vi "Test Functionality.vi"() -> ()   [LabVIEW 2013, in "Exponential Fit Library.lvlib" / "Fit Exponential.lvclass"]
doc: "This is a simle demonstration of the capabilities of the exponential fit class."
uses:
  Fit Exponential.lvclass
  Fit Exponential.lvclass/Fit Exponential.ctl
  Children/DFT-1/DFT-1.lvclass
  Children/DFT-5/DFT-5.lvclass
  Children/LRS/LRS.lvclass
  Read Output.vi
  <vilib>/Analysis/1siggen.llb/Ramp Pattern by Delta.vi
  <vilib>/Analysis/NI_AALBase.lvlib
panel:
  out "Fit Output":T1
  in  "B":dbl
  in  "A":dbl
  in  "tau":dbl
  in  "Select Method":enum8{"DFT-1", "DFT-5", "LRS"}(ring)=enum."LRS"
  out "Error in Tau":dbl(graph)
  out "Tau":dbl(graph)
  out "Exponential":dbl[](graph)
  # "Exponential Input"
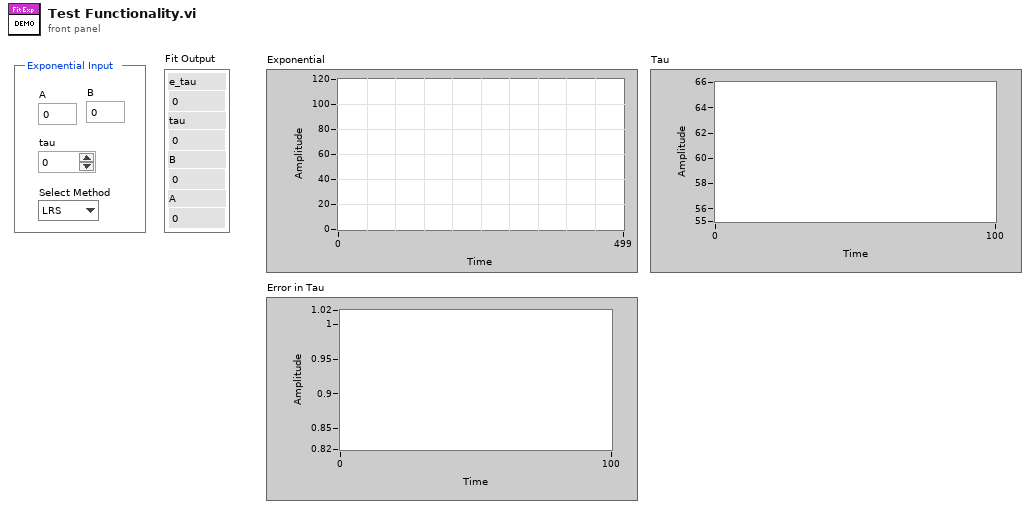
[diagram p1: front panel]
types:
  T1 = cluster{"e_tau":dbl, "tau":dbl, "B":dbl, "A":dbl}
  T2 = cluster{"A":dbl, "B":dbl, "tau":dbl, "e_tau":dbl}
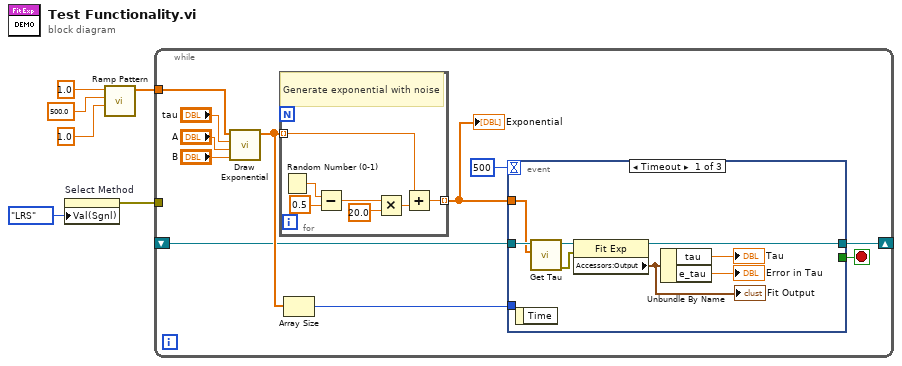
[diagram p0: block diagram]
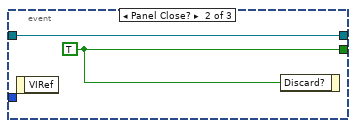
[diagram p2: hidden frame]
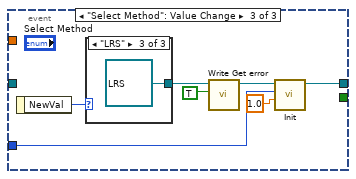
[diagram p3: hidden frame]
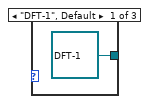
[diagram p4: hidden frame]
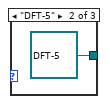
[diagram p5: hidden frame]
diagram:
  n1 = property on="Select Method" class="Enum (strict)"("Val(Sgnl)"=enum8{"DFT-1", "DFT-5", "LRS"}."LRS" ("Value (Signaling)")) -> (error out=w1:errorcluster)  [unwired: 2 in, 1 out]
  n2 = call-poly <vilib>:"Ramp Pattern.vi"("start"=1.0, "end"=500.0, "delta"=1.0) -> ("Ramp Pattern"=w3:dbl[])  [unwired: 6 in, 2 out]
  n3 = while {
    tunnel: w3 -> [w17]
    shift-right: [w13] -> _
    shift-left: _ -> [w9]
    tunnel: w1 -> [_]
    stop <- w7 stop-if-true
    n4 = call "Draw Exponential.vi"("B"="B", "A"="A", "tau"="tau", "time"=w17) -> ("ExponentialOut"=w12:dbl[])  [unwired: 7 in]
    n5 = for {
      tunnel: w12 -> [w39] mode=indexing
      tunnel: [w38] -> w8 mode=indexing
      # "Generate exponential with noise"
      n6 = Random Number (0-1)() -> (number: 0 to 1=w44:dbl)
      n7 = Subtract(x=w44, y=0.5) -> (x-y=w42:dbl)
      n8 = Multiply(x=w42, y=20.0) -> (x*y=w40:dbl)
      n9 = Add(x=w39, y=w40) -> (x+y=w38:dbl)
    }
    "Exponential" <- w8
    n10 = Array Size(array=w12) -> (size(s)=w11:i32)
    n11 = event shown="[0] Timeout" {
      selector: _ -> [_ _ _]
      dyn-events: _ -> [_ _ _]
      timeout: 500 -> [_ _ _]
      tunnel: [w22 w26 w33] -> w13
      tunnel: w11 -> [_ _ w32]
      tunnel: w9 -> [w25 w26 _]
      tunnel: w8 -> [w21 _ _]
      tunnel: [_ w27 _] -> w7
      event Timeout {
        n12 = event-data() -> ()  [unwired: 1 in, 1 out]
        n13 = call "Get Tau.vi"("Data In"=w21, "Fit Exp in"=w25) -> ("error out"=w23:errorcluster, "Fit Exp out"=w24:refnum<class "Fit Exponential.lvclass">)  [unwired: 8 in]
        n14 = property class="Fit Exp"(reference=w24, error in=w23) -> (reference out=w22:refnum<class "Fit Exponential.lvclass">, "Accessors:Output"=w18:T2)  [unwired: 1 out]
        "Fit Output" <- w18
        n15 = Unbundle By Name(w18) -> ("tau"=→"Tau":dbl, "e_tau"=→"Error in Tau":dbl)
      }
      event Panel Close? {
        w27 = TRUE
        n16 = event-data() -> ()  [unwired: 1 in, 1 out]
        n17 = event-data("Discard?"=w27) -> ()  [unwired: 1 in, 1 out]
      }
      event "Select Method": Value Change {
        n18 = event-data() -> ("NewVal"=w34:enum8{"DFT-1", "DFT-5", "LRS"})  [unwired: 1 in]
        n19 = case shown="\"LRS\"" w34 {
          tunnel: [refnum<class "DFT-1.lvclass"> refnum ("Exponential Fit Library.lvlib:DFT-1") refnum<class "DFT-5.lvclass"> refnum ("Exponential Fit Library.lvlib:DFT-5") refnum<class "LRS.lvclass"> refnum ("Exponential Fit Library.lvlib:LRS")] -> w30
          frame "DFT-1", Default {
          }
          frame "DFT-5" {
          }
          frame "LRS" {
          }
        }
        n20 = call "Write Get error.vi"("Get error?"=TRUE, "Fit Exponential in"=w30) -> ("Fit Exponential out"=w29:refnum<class "Fit Exponential.lvclass">)  [unwired: 8 in, 1 out]
        n21 = call-dynamic "Init.vi"("Dt"=1.0, "Size"=w32, "Fit Exponential in"=w29) -> ("Fit Exponential out"=w33:refnum<class "Fit Exponential.lvclass">)  [unwired: 8 in]
      }
    }
  }
